vi "WLAN_FrameCapture.vi"(7 "error in (no error)":errorcluster, 9 "Trigger level":dbl format="%0.2f", 10 "session handle":refnum<k15>) -> ()   [LabVIEW 2022 SP3]
uses:
  <instrlib>/niUSRP/niUSRP Fetch Rx Data (CDB Cluster).vi
  <vilib>/Analysis/NI_AALPro.lvlib
panel:
  out "error out":errorcluster
  out "Waveform Graph":cluster{"t0":dbl, "dt":dbl, "Y":dbl[]}(graph)
  out "x <= y?":bool
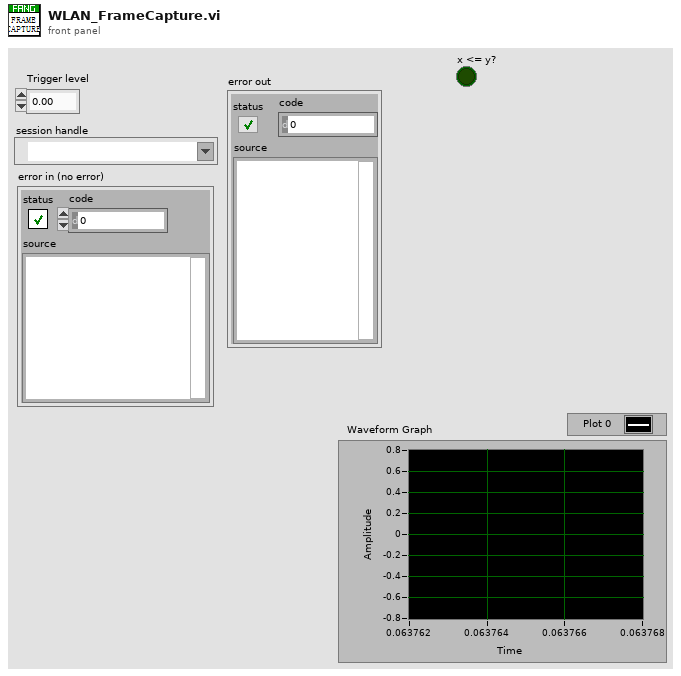
[diagram p1: front panel]
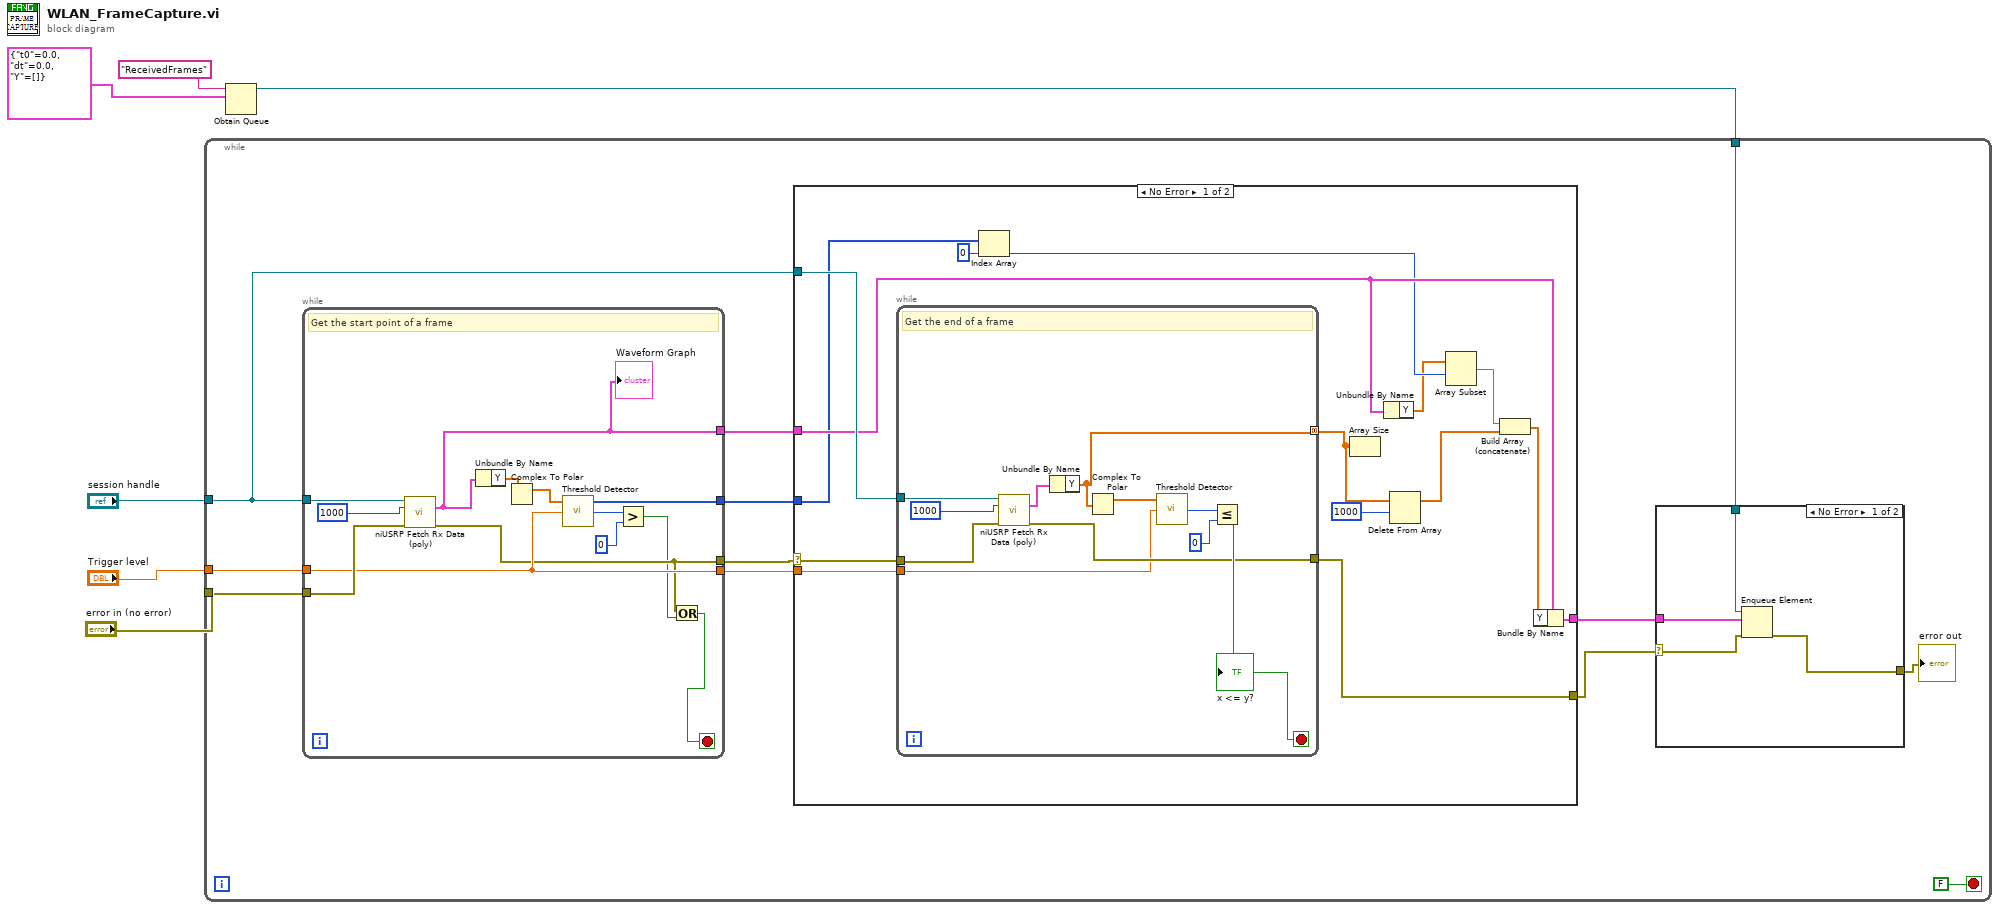
[diagram p0: block diagram]
diagram:
  n1 = Obtain Queue(name (unnamed)="ReceivedFrames", element data type=cluster{"t0":dbl, "dt":dbl, "Y":cdb[]} {"t0"=0.0, "dt"=0.0, "Y"=[]} ("data")) -> (queue out=w1:refnum<queue>)  [unwired: 3 in, 2 out]
  n2 = while {
    tunnel: "error in (no error)" -> [w18]
    tunnel: "Trigger level" -> [w17]
    tunnel: "session handle" -> [w16]
    tunnel: w1 -> [w11]
    stop <- FALSE stop-if-true
    n3 = while {
      tunnel: w16 -> [w61]
      tunnel: w18 -> [w64]
      tunnel: w17 -> [w59]
      tunnel: [w54] -> w12
      tunnel: [w59] -> w15
      tunnel: [w55] -> w14
      tunnel: [w56] -> w13
      stop <- w52 stop-if-true
      # "Get the start point of a frame"
      n4 = call-poly <instrlib>:"niUSRP Fetch Rx Data (poly).vi"("session handle"=w61, "number of samples"=i64 1000, "error in (no error)"=w64) -> ("data"=w55:cluster{"t0":dbl, "dt":dbl, "Y":cdb[]}, "error out"=w54:errorcluster)  [unwired: 9 in, 2 out]
      "Waveform Graph" <- w55
      n5 = Unbundle By Name(w55) -> ("Y"=w57:cdb[])
      n6 = Complex To Polar(r * e^(i*theta)=w57) -> (r=w58:dbl[])  [unwired: 1 out]
      n7 = call <vilib>:"Threshold Detector.vi"("threshold"=w59, "X"=w58) -> ("count"=w63:i32, "Indices"=w56:i32[])  [unwired: 1 in, 1 out]
      n8 = Greater?(x=w63, y=0) -> (0:w53:bool)
      n9 = Or(x=w54, y=w53) -> (x .or. y?=w52:bool)
    }
    n10 = case shown="No Error" w12 {
      selector: w12 -> [w24 w50]
      tunnel: w16 -> [w38 _]
      tunnel: [w37 w50] -> w9
      tunnel: w15 -> [w36 _]
      tunnel: w14 -> [w35 w51]
      tunnel: [w34 w51] -> w10
      tunnel: w13 -> [w29 _]
      frame No Error {
        n11 = while {
          tunnel: w38 -> [w47]
          tunnel: [w44] -> w37
          tunnel: w24 -> [w43]
          tunnel: w36 -> [w42]
          tunnel: [w39] -> w33 mode=concatenating
          stop <- w45 stop-if-true
          # "Get the end of a frame"
          n12 = call-poly <instrlib>:"niUSRP Fetch Rx Data (poly).vi"("session handle"=w47, "number of samples"=i64 1000, "error in (no error)"=w43) -> ("data"=w40:cluster{"t0":dbl, "dt":dbl, "Y":cdb[]}, "error out"=w44:errorcluster)  [unwired: 9 in, 2 out]
          n13 = Unbundle By Name(w40) -> ("Y"=w39:cdb[])
          n14 = Complex To Polar(r * e^(i*theta)=w39) -> (r=w41:dbl[])  [unwired: 1 out]
          n15 = call <vilib>:"Threshold Detector.vi"("threshold"=w42, "X"=w41) -> ("count"=w49:i32)  [unwired: 1 in, 2 out]
          n16 = Less Or Equal?(x=w49, y=0) -> (x <= y?=w45:bool)
          "x <= y?" <- w45
        }
        n17 = Index Array(array=w29, index=0) -> (element=w27:i32)
        n18 = Array Size(array=w33) -> ()  [unwired: 1 out]
        n19 = Unbundle By Name(w35) -> ("Y"=w26:cdb[])
        n20 = Delete From Array(array=w33, length=1000) -> (array with subset deleted=w31:cdb[])  [unwired: 1 in, 1 out]
        n21 = Array Subset(array=w26, index=w27) -> (w25:cdb[])  [unwired: 1 in]
        n22 = Build Array (concatenate)(w25, w31) -> (w30:cdb[])
        n23 = Bundle By Name(cluster=w35, "Y"=w30) -> (w34:cluster{"t0":dbl, "dt":dbl, "Y":cdb[]})
      }
      frame Error {
      }
    }
    n24 = case shown="No Error" w9 {
      selector: w9 -> [w20 w23]
      tunnel: w11 -> [w22 _]
      tunnel: w10 -> [w21 _]
      tunnel: [w19 w23] -> w8
      frame No Error {
        n25 = Enqueue Element(queue=w22, element=w21, error in (no error)=w20) -> (error out=w19:errorcluster)  [unwired: 1 in, 2 out]
      }
      frame Error {
      }
    }
    "error out" <- w8
  }
